vi "load_array_of_boxes_xml.vi"(8 "error in":errorcluster, 11 "node result array":refnum<k20>[](array[refnum])) -> (0 "error out":errorcluster, 3 "ArrayOfDDSBoxes":T1[](array[typedef]) {"Array of DDS Channels (4)"."Channel Parameters"."Ref Clock Rate [kHz]" min=0.0})   [LabVIEW 2013, in "DDS.lvclass"]
doc: "Loads array of DDS boxes from XML. Expected format:\n\n<box>\n<Enable>%b</Enable>\n<DDSBoxDeviceReference.Resource>%s</DDSBoxDeviceReference.Resource>\n<DDSBoxDeviceReference.DIOPort>%u</DDSBoxDeviceReference.DIOPort>\n<DDSBoxDeviceReference.SerialClockRate units=\"kHz\">%u</DDSBoxDeviceReference.SerialClockRate>\n<ArrayOfDDSChannels>\n\n<channel>\n<Power>%b</Power>\n<ChannelParameters.RefClockRate units=\"kHz\">%f</ChannelParameters.RefClockRate>\n<ChannelParameters.FullScaleOutputPower units=\"dBm\">%f</ChannelParameters.FullScaleOutputPower>\n<RAMEnable>%b</RAMEnable>\n<RAMDestType>%u</RAMDestType>\n<RAMDefault.Frequency units=\"MHz\">%s</RAMDefault.Frequency>\n<RAMDefault.Amplitude units=\"dBm\">%s</RAMDefault.Amplitude>\n<RAMDefault.Phase units=\"rad\">%s</RAMDefault.Phase>\n<ArrayOfDDSProfiles>\n\n<profile>\n<SingleTone.Frequency units=\"MHz\">%s</SingleTone.Frequency>\n<SingleTone.Amplitude units=\"dBm\">%s</SingleTone.Amplitude>\n<SingleTone.Phase units=\"rad\">%s</SingleTone.Phase>\n<RAMMode>%u</RAMMode>\n<ZeroCrossing>%b</ZeroCrossing>\n<NoDwellHigh>%b</NoDwellHigh>\n<FunctionOrStatic>%b</FunctionOrStatic>\n<RAMFunctionSettings>%s</RAMFunctionSettings>\n<RAMStaticArray>%s</RAMStaticArray>\n</profile>\n\n</ArrayOfDDSProfiles>\n</channel>\n\n</ArrayOfDDSChannels>\n</box>\n\nMTL 2012 Dec 31"
uses:
  DDS.lvclass
  DDS drivers v3/DDS_box_cluster.ctl
  DDS drivers v3/DDS_box_device_reference.ctl
  <vilib>/ni845x/ni845x.llb/ni845xControl.ctl
  DDS drivers v3/array_of_DDS_channels.ctl
  DDS drivers v3/DDS_channel.ctl
  DDS drivers v3/array_of_DDS_profiles.ctl
  DDS drivers v3/DDS_profile.ctl
  DDS drivers v3/DDS RAM mode.ctl
  <vilib>/xml/Close Reference(Node).vi
  <resource>/objmgr/DOMUserDefRef.rc
  <vilib>/xml/NI_XML.lvlib
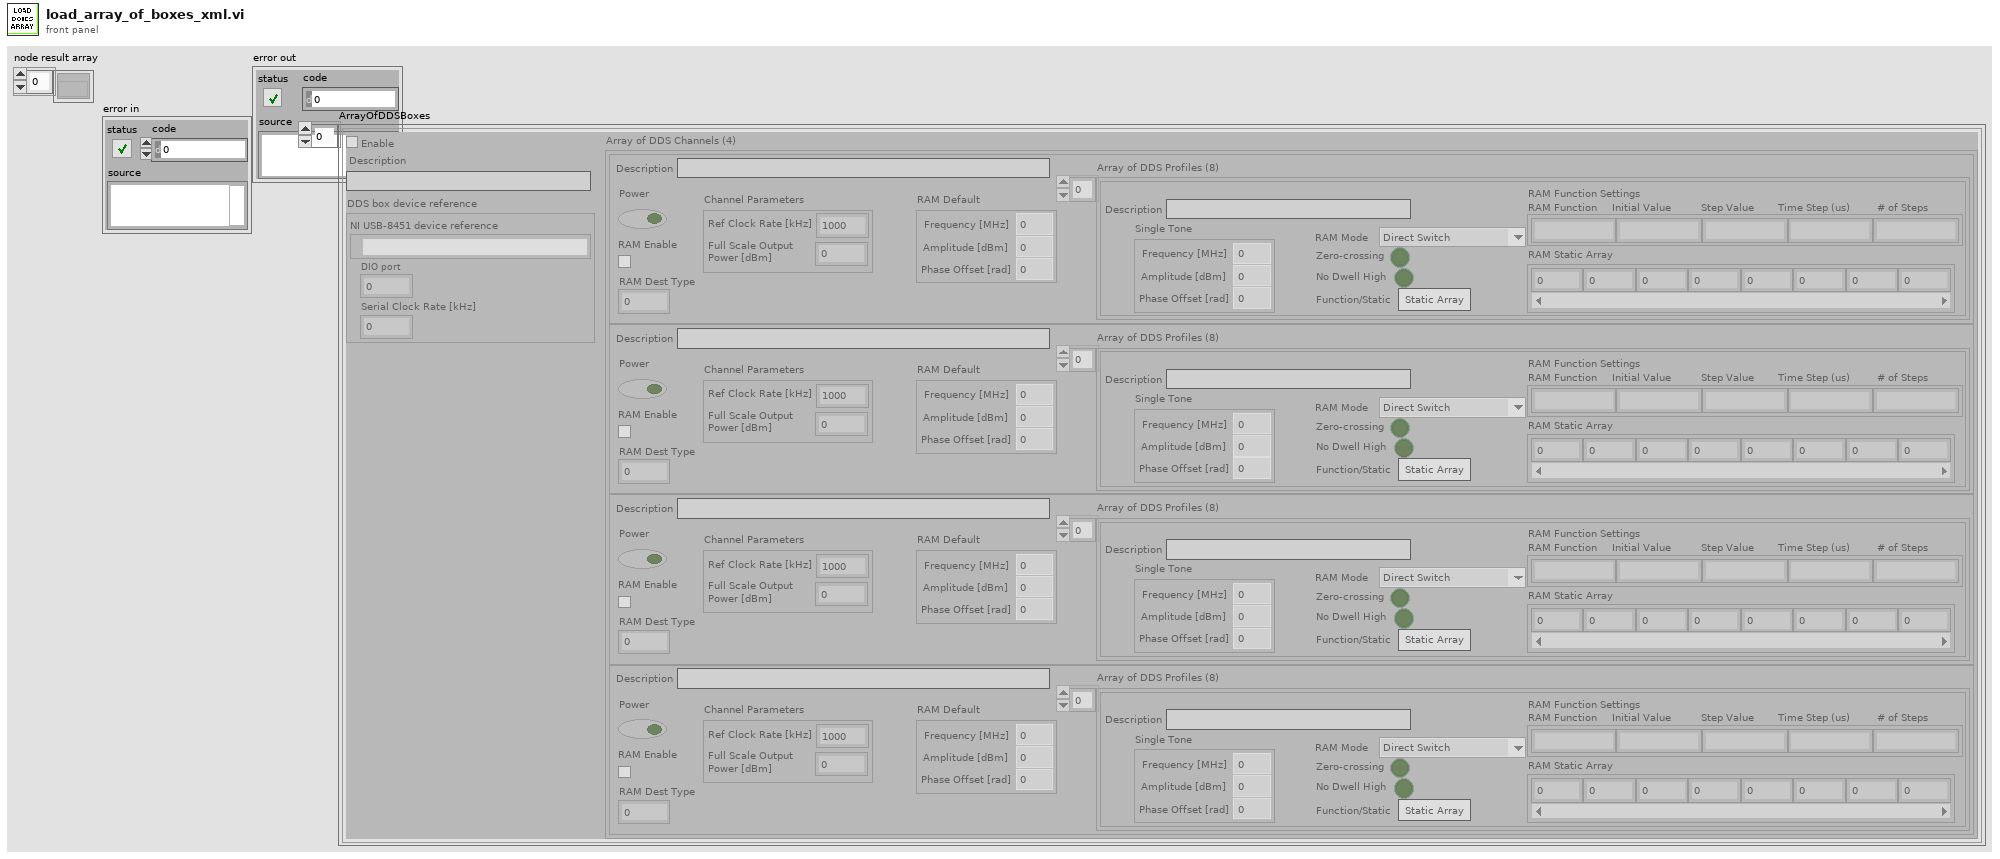
[diagram p1: front panel]
types:
  T1 = typedef "DDS_box_cluster.ctl" = cluster{"DDS box device reference":T2, "Array of DDS Channels (4)":T4, "Enable":bool, "Description":string}
  T2 = typedef "DDS_box_device_reference.ctl" = cluster{"NI USB-8451 device reference":T3, "DIO port":u8, "Serial Clock Rate [kHz]":u16}
  T3 = typedef "ni845xControl.ctl" = refnum<k21>
  T4 = typedef "DDS.lvclass/array_of_DDS_channels.ctl" = T5[]
  T5 = typedef "DDS.lvclass/DDS_channel.ctl" = cluster{"Power":bool, "Channel Parameters":cluster{"Ref Clock Rate [kHz]":dbl, "Full Scale Output\nPower [dBm]":dbl}, "RAM Enable":bool, "RAM Dest Type":u8, "RAM Default":cluster{"Frequency [MHz]":dbl, "Amplitude [dBm]":dbl, "Phase Offset [rad]":dbl}, "Array of DDS Profiles (8)":T6, "Description":string}
  T6 = typedef "DDS.lvclass/array_of_DDS_profiles.ctl" = T7[]
  T7 = typedef "DDS_profile.ctl" = cluster{"Single Tone":cluster{"Frequency [MHz]":dbl, "Amplitude [dBm]":dbl, "Phase Offset [rad]":dbl}, "RAM Mode ":T8, "Zero-crossing":bool, "No Dwell High":bool, "Function/Static":bool, "RAM Function Settings":string[], "RAM Static Array":dbl[], "Description":string}
  T8 = typedef "DDS RAM mode.ctl" = enum16{"Direct Switch", "Ramp Up", "Bidirectional Ramp", "Continuous Bidirectional Ramp", "Continuous Recirculate", "Direct Switch 2", "Direct Switch 3", "Direct Switch 4"}
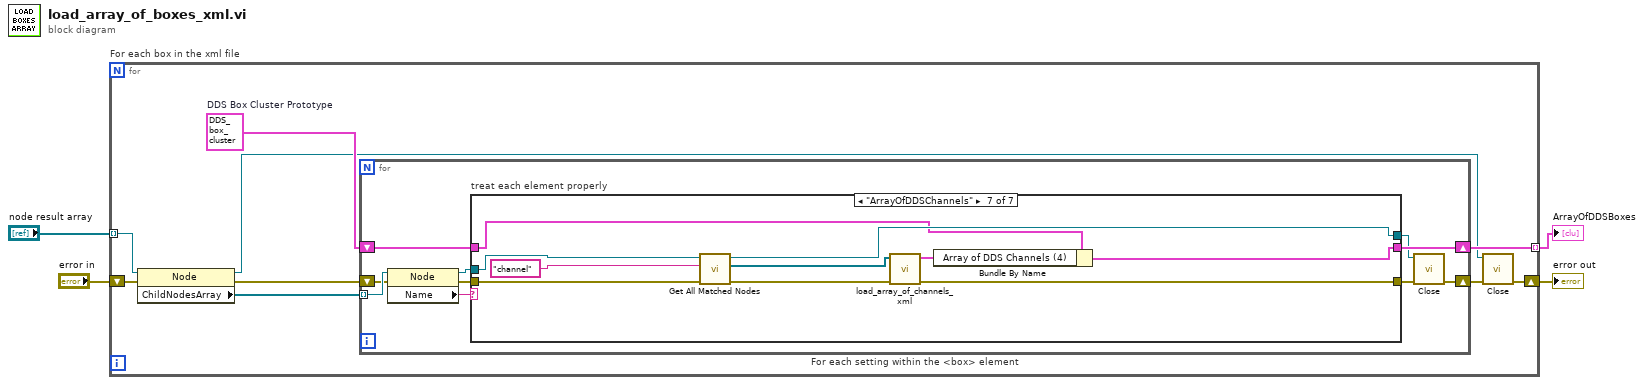
[diagram p0: block diagram]
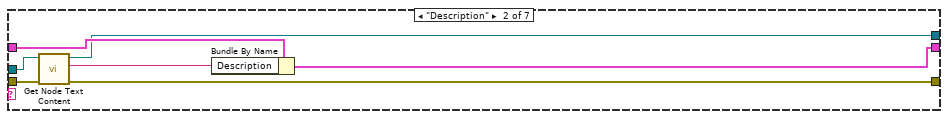
[diagram p3: hidden frame]
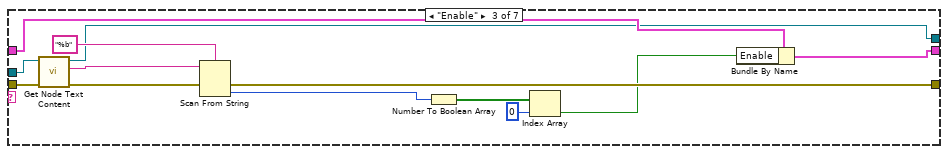
[diagram p4: hidden frame]
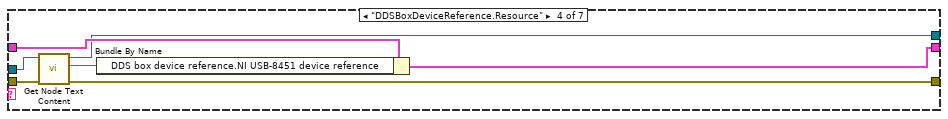
[diagram p5: hidden frame]
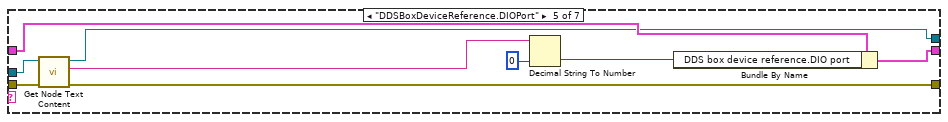
[diagram p6: hidden frame]
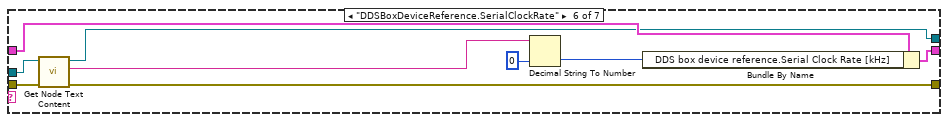
[diagram p7: hidden frame]
diagram:
  n1 = for "For each box in the xml file" {
    tunnel: "node result array" -> [w11] mode=indexing
    shift-right: [w5] -> w2
    shift-left: "error in" -> [w10]
    tunnel: [w13] -> w1 mode=indexing
    w12 = T1 {"DDS box device reference"={"NI USB-8451 device reference"="USB0::0x3923::0x7166::0166CE36::RAW", "DIO port"=0, "Serial Clock Rate [kHz]"=1000}, "Array of DDS Channels (4)"=[{"Power"=FALSE, "Channel Parameters"={"Ref Clock Rate [kHz]"=0.0, "Full Scale Output\nPower [dBm]"=0.0}, "RAM Enable"=FALSE, "RAM Dest Type"=0, "RAM Default"={"Frequency [MHz]"=0.0, "Amplitude [dBm]"=0.0, "Phase Offset [rad]"=0.0}, "Array of DDS Profiles (8)"=[], "Description"=""}, {"Power"=FALSE, "Channel Parameters"={"Ref Clock Rate [kHz]"=0.0, "Full Scale Output\nPower [dBm]"=0.0}, "RAM Enable"=FALSE, "RAM Dest Type"=0, "RAM Default"={"Frequency [MHz]"=0.0, "Amplitude [dBm]"=0.0, "Phase Offset [rad]"=0.0}, "Array of DDS Profiles (8)"=[], "Description"=""}, {"Power"=FALSE, "Channel Parameters"={"Ref Clock Rate [kHz]"=0.0, "Full Scale Output\nPower [dBm]"=0.0}, "RAM Enable"=FALSE, "RAM Dest Type"=0, "RAM Default"={"Frequency [MHz]"=0.0, "Amplitude [dBm]"=0.0, "Phase Offset [rad]"=0.0}, "Array of DDS Profiles (8)"=[], "Description"=""}, {"Power"=FALSE, "Channel Parameters"={"Ref Clock Rate [kHz]"=0.0, "Full Scale Output\nPower [dBm]"=0.0}, "RAM Enable"=FALSE, "RAM Dest Type"=0, "RAM Default"={"Frequency [MHz]"=0.0, "Amplitude [dBm]"=0.0, "Phase Offset [rad]"=0.0}, "Array of DDS Profiles (8)"=[], "Description"=""}], "Enable"=FALSE, "Description"=""}  # DDS Box Cluster Prototype
    n2 = property class="Node"(reference=w11, error in=w10) -> (reference out=w7:refnum<k20>, error out=w8:errorcluster, "ChildNodesArray"=w9:refnum<k20>[])
    n3 = for "For each setting within the <box> element" {
      shift-right: [w21] -> w13
      shift-left: w12 -> [w20]
      tunnel: w9 -> [w19] mode=indexing
      shift-right: [w23] -> w6
      shift-left: w8 -> [w18]
      n4 = property class="Node"(reference=w19, error in=w18) -> (reference out=w15:refnum<k20>, error out=w16:errorcluster, "Name"=w17:string)
      n5 = case "treat each element properly" shown="\"ArrayOfDDSChannels\"" w17 {
        tunnel: w16 -> [w26 w30 w37 w50 w55 w66 w78]
        tunnel: [w26 w29 w42 w49 w54 w65 w73] -> w22
        tunnel: w20 -> [w25 w33 w41 w53 w62 w71 w77]
        tunnel: [w25 w32 w39 w52 w61 w70 w76] -> w21
        tunnel: w15 -> [w24 w31 w38 w51 w58 w67 w80]
        tunnel: [w24 w28 w35 w48 w57 w64 w79] -> w14
        frame "None", Default {
        }
        frame "Description" {
          n6 = call <vilib>:"Get Node Text Content.vi"("error in (no error)"=w30, "node in"=w31) -> ("error out"=w29:errorcluster, "node text"=w27:string, "node out"=w28:refnum<k20>)  [unwired: 7 in]
          n7 = Bundle By Name(cluster=w33, "Description"=w27) -> (w32:T1)
        }
        frame "Enable" {
          n8 = call <vilib>:"Get Node Text Content.vi"("error in (no error)"=w37, "node in"=w38) -> ("error out"=w36:errorcluster, "node text"=w34:string, "node out"=w35:refnum<k20>)  [unwired: 7 in]
          n9 = Scan From String(format string="%b", input string=w34, error in=w36) -> (error out=w42:errorcluster, output 1=w43:i32)  [unwired: 2 in, 2 out]
          n10 = Number To Boolean Array(number=w43) -> (Boolean array=w46:bool[])
          n11 = Index Array(array=w46, index=0) -> (element=w40:bool)
          n12 = Bundle By Name(cluster=w41, "Enable"=w40) -> (w39:T1)
        }
        frame "DDSBoxDeviceReference.Resource" {
          n13 = call <vilib>:"Get Node Text Content.vi"("error in (no error)"=w50, "node in"=w51) -> ("error out"=w49:errorcluster, "node text"=w47:string, "node out"=w48:refnum<k20>)  [unwired: 7 in]
          n14 = Bundle By Name(cluster=w53, "DDS box device reference.NI USB-8451 device reference"=w47) -> (w52:T1)
        }
        frame "DDSBoxDeviceReference.DIOPort" {
          n15 = call <vilib>:"Get Node Text Content.vi"("error in (no error)"=w55, "node in"=w58) -> ("error out"=w54:errorcluster, "node text"=w56:string, "node out"=w57:refnum<k20>)  [unwired: 7 in]
          n16 = Decimal String To Number(string=w56, default (0L)=u8 0 ("default (0 I32)")) -> (number=w59:u8)  [unwired: 1 in, 1 out]
          n17 = Bundle By Name(cluster=w62, "DDS box device reference.DIO port"=w59) -> (w61:T1)
        }
        frame "DDSBoxDeviceReference.SerialClockRate" {
          n18 = call <vilib>:"Get Node Text Content.vi"("error in (no error)"=w66, "node in"=w67) -> ("error out"=w65:errorcluster, "node text"=w63:string, "node out"=w64:refnum<k20>)  [unwired: 7 in]
          n19 = Decimal String To Number(string=w63, default (0L)=u16 0 ("default (0 I32)")) -> (number=w69:u16)  [unwired: 1 in, 1 out]
          n20 = Bundle By Name(cluster=w71, "DDS box device reference.Serial Clock Rate [kHz]"=w69) -> (w70:T1)
        }
        frame "ArrayOfDDSChannels" {
          n21 = call <vilib>:"Get All Matched Nodes.vi"("error in (no error)"=w78, "XPath expression"="channel", "node in"=w80) -> ("error out"=w75:errorcluster, "node result array"=w74:refnum<k20>[], "node out"=w79:refnum<k20>)  [unwired: 6 in]
          n22 = call "load_array_of_channels_xml.vi"("error in"=w75, "node result array"=w74) -> ("error out"=w73:errorcluster, "Array of DDS Channels (4)"=w72:T4)  [unwired: 8 in]
          n23 = Bundle By Name(cluster=w77, "Array of DDS Channels (4)"=w72) -> (w76:T1)
        }
      }
      n24 = call-poly <vilib>:"Close.vi"("error in (no error)"=w22, "node"=w14) -> ("error out"=w23:errorcluster)  [unwired: 7 in]
    }
    n25 = call-poly <vilib>:"Close.vi"("error in (no error)"=w6, "node"=w7) -> ("error out"=w5:errorcluster)  [unwired: 7 in]
  }
  "error out" <- w2
  "ArrayOfDDSBoxes" <- w1
